vi "picoharp_write_user_events.vi"(7 "update_hydraharp_status":refnum<user-event>, 8 "error in (no error)":errorcluster, 10 "ui_events":T1, 11 "hydraharp in":refnum<class "picoharp.lvclass">) -> (0 "error out":errorcluster, 3 "hydraharp out":refnum<class "picoharp.lvclass">)   [LabVIEW 2015, in "picoharp.lvclass"]
uses:
  picoharp.lvclass
  UI/front_panel_class/ui_user_events.ctl
  Hydraharp/hydraharp/hydraharp_user_events.ctl
  picoharp.lvclass/picoharp.ctl
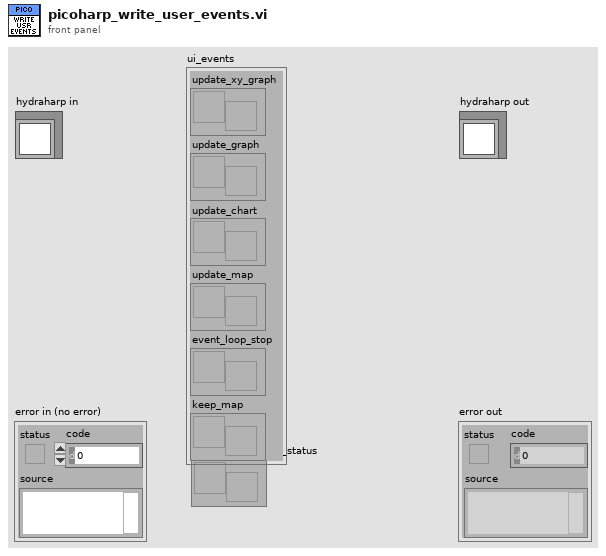
[diagram p1: front panel]
types:
  T1 = typedef "ui_user_events.ctl" = cluster{"update_xy_graph":refnum<user-event>, "update_graph":refnum<user-event>, "update_chart":refnum<user-event>, "update_map":refnum<user-event>, "event_loop_stop":refnum<user-event>, "keep_map":refnum<user-event>}
  T2 = typedef "hydraharp_user_events.ctl" = cluster{"ui_events":T1, "update_hydraharp_status":refnum<user-event>}
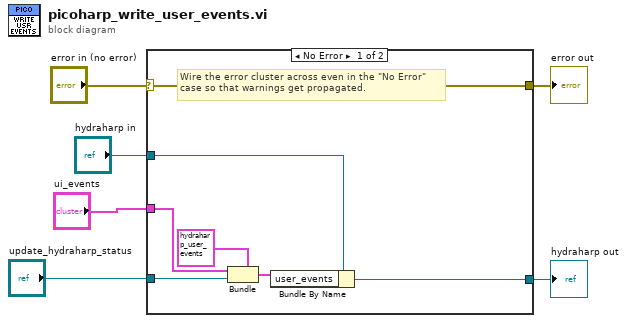
[diagram p0: block diagram]
diagram:
  n1 = case shown="No Error" "error in (no error)" {
    selector: "error in (no error)" -> [w13 w15]
    tunnel: [w13 w15] -> w5
    tunnel: [w8 w14] -> w3
    tunnel: "hydraharp in" -> [w9 w14]
    tunnel: "ui_events" -> [w12 _]
    tunnel: "update_hydraharp_status" -> [w11 _]
    frame No Error {
      # "Wire the error cluster across even in the \"No Error\"\ncase so that warnings get propagated."
      n2 = Bundle(cluster=T2 {"ui_events"={"update_xy_graph"=refnum, "update_graph"=refnum, "update_chart"=refnum, "update_map"=refnum, "event_loop_stop"=refnum, "keep_map"=refnum}, "update_hydraharp_status"=refnum} ("output cluster"), "ui_events"=w12, "update_hydraharp_status"=w11) -> (w7:T2)
      n3 = Bundle By Name(cluster=w9, "user_events"=w7) -> (w8:refnum<class "picoharp.lvclass">)
    }
    frame Error {
    }
  }
  "error out" <- w5
  "hydraharp out" <- w3
